vi "离线数据源.vi"(11 "显示前面板":bool) -> (0 "前面板打开":bool, 1 "电流":dbl[](array[numeric]), 2 "电压数据":dbl[](array[numeric]), 3 "脉冲数据":u32[](array[numeric]))   [LabVIEW 2020]
uses:
  <vilib>/Analysis/baseanly.llb/Mean (DBL).vi
  TCPModbus_MasterClient/MB Ethernet Master Query Read Input Registers (poly).vi
  <vilib>/Analysis/NI_AALBase.lvlib
panel:
  in  "噪声比例":dbl(knob)=0.01 min=0.01 max=0.99 step=0.01 scale=0.01..0.99 scale format="%#.2f"
  in  "加载白噪声":bool
  in  "P2-7":u16(ring)=1 items=["源量程计数CPS", "中间量程电流A", "棒位STEP", "温度(摄氏度)", "硼浓度PPM", "P2电压信号"]
  in  "P2-6":u16(ring)=1 items=["源量程计数CPS", "中间量程电流A", "棒位STEP", "温度(摄氏度)", "硼浓度PPM", "P2电压信号"]
  in  "P2-8":u16(ring) items=["源量程计数CPS", "中间量程电流A", "棒位STEP", "温度(摄氏度)", "硼浓度PPM", "P2电压信号"]
  in  "P2-5":u16(ring)=4 items=["源量程计数CPS", "中间量程电流A", "棒位STEP", "温度(摄氏度)", "硼浓度PPM", "P2电压信号"]
  in  "P2-4":u16(ring)=3 items=["源量程计数CPS", "中间量程电流A", "棒位STEP", "温度(摄氏度)", "硼浓度PPM", "P2电压信号"]
  in  "P2-3":u16(ring)=5 items=["源量程计数CPS", "中间量程电流A", "棒位STEP", "温度(摄氏度)", "硼浓度PPM", "P2电压信号"]
  in  "P2-2":u16(ring)=2 items=["源量程计数CPS", "中间量程电流A", "棒位STEP", "温度(摄氏度)", "硼浓度PPM", "P2电压信号"]
  in  "P2-6":dbl=3e-12
  in  "P2-5":dbl=500.0
  in  "P2-4":dbl=275.0
  in  "P2-3":dbl
  in  "P2-1":u16(ring)=2 items=["源量程计数CPS", "中间量程电流A", "棒位STEP", "温度(摄氏度)", "硼浓度PPM", "P2电压信号"]
  out "TCP Connection":refnum<k5>
  in  "网络端口":u16=502
  in  "网络连接IP地址":string="192.168.1.66"
  in  "网络数据源开":bool
  in  "网络数据源开关":bool
  in  "1-5V":bool
  out "Vin8":dbl format="%#_5g"
  out "Vin7":dbl format="%#_5g"
  out "Vin6":dbl format="%#_5g"
  out "Vin5":dbl format="%#_5g"
  out "Vin4":dbl format="%#_5g"
  out "Vin3":dbl format="%#_5g"
  out "Vin2":dbl format="%#_5g"
  out "Vin1":dbl format="%#_5g"
  in  "电流通道2":dbl=2e-11
  in  "电流通道1":dbl=1e-11
  in  "P2-8":dbl=1.0
  in  "P2-7":dbl=4e-12
  in  "P2-2":dbl
  in  "P2-1":dbl
  in  "脉冲3":u32=300
  in  "脉冲2":u32=200
  in  "脉冲1":u32=100
  # "CPS"
  # "A"
  # "CPS"
  # "A"
  # "CPS"
  # "0-10V"
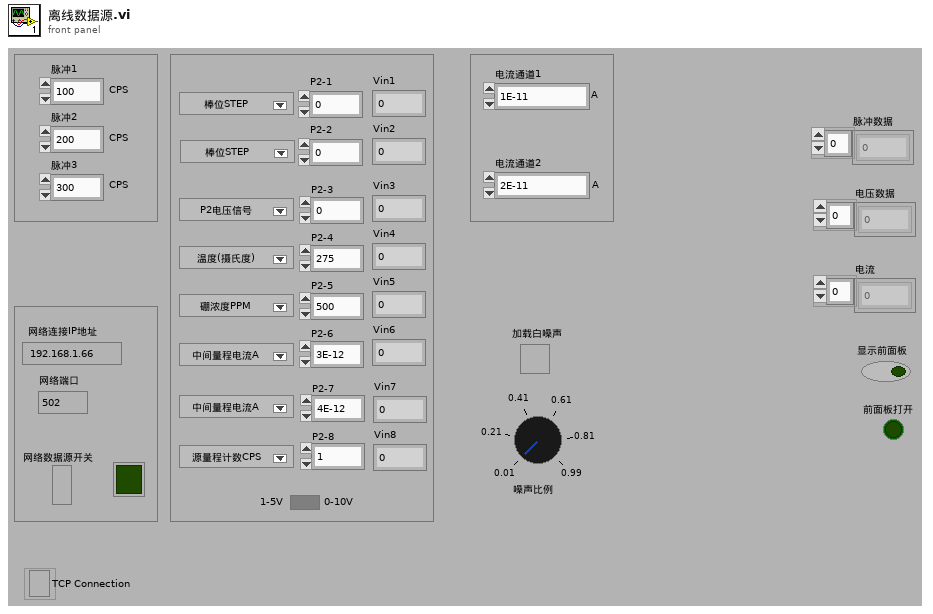
[diagram p1: front panel]
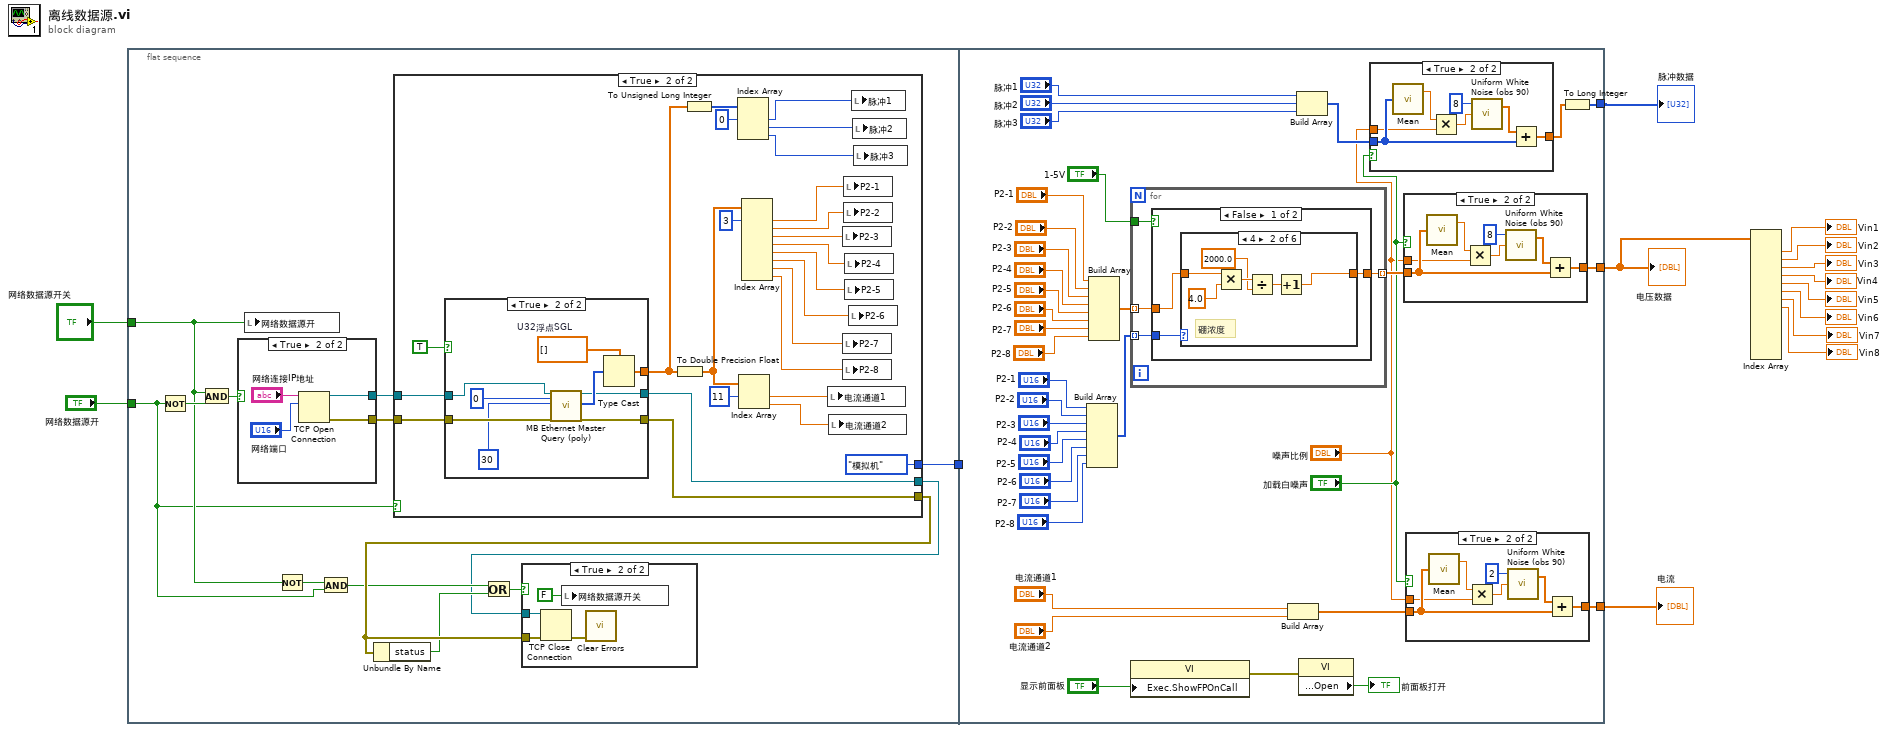
[diagram p0: block diagram]
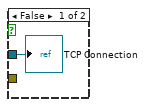
[diagram p2: hidden frame]
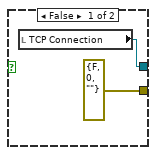
[diagram p3: hidden frame]
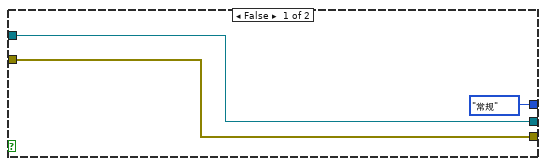
[diagram p4: hidden frame]
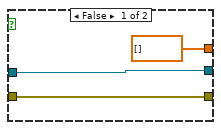
[diagram p5: hidden frame]
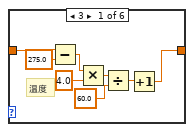
[diagram p9: hidden frame]
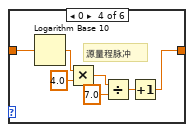
[diagram p11: hidden frame]
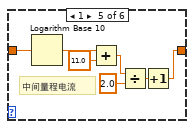
[diagram p12: hidden frame]
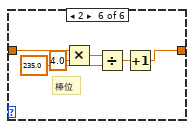
[diagram p13: hidden frame]
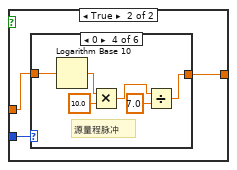
[diagram p14: hidden frame]
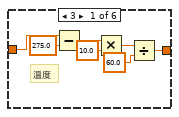
[diagram p15: hidden frame]
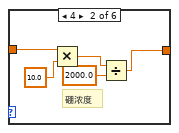
[diagram p16: hidden frame]
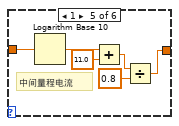
[diagram p18: hidden frame]
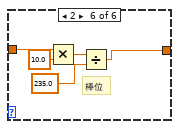
[diagram p19: hidden frame]
diagram:
  n1 = flat-sequence {
    tunnel: "网络数据源开关" -> [w24]
    tunnel: [w27] -> w13
    tunnel: "网络数据源开" -> [w22]
    tunnel: [w85] -> w3
    tunnel: [w87] -> w1
    tunnel: [w82] -> w2
    tunnel: w13 -> [_]
    frame #0 {
      n2 = Not(x=w22) -> (.not. x?=w26:bool)
      n3 = And(x=w24, y=w26) -> (x .and. y?=w25:bool)
      n4 = case shown="True" w25 {
        tunnel: [w33 w36] -> w21
        tunnel: [errorcluster {"status"=FALSE, "code"=0, "source"=""} ("error out") w35] -> w20
        frame False {
          n5 = local read "TCP Connection"() -> (w33:refnum<k5>)
        }
        frame True {
          n6 = TCP Open Connection(address="网络连接IP地址", remote port or service name="网络端口") -> (connection ID=w36:refnum<k5>, error out=w35:errorcluster)  [unwired: 1 in, 2 out]
        }
      }
      n7 = local write "网络数据源开"(w24) -> ()
      n8 = Not(x=w24) -> (.not. x?=w23:bool)
      n9 = And(x=w23, y=w22) -> (x .and. y?=w18:bool)
      n10 = case shown="True" w22 {
        tunnel: [enum32{"常规", "模拟机"}."常规" ("选项") enum32{"常规", "模拟机"}."模拟机" ("选项")] -> w27
        tunnel: w21 -> [w40 w52]
        tunnel: w20 -> [w39 w51]
        tunnel: [w39 w48] -> w19
        tunnel: [w40 w49] -> w15
        frame False {
        }
        frame True {
          n11 = case shown="True" TRUE {
            tunnel: w52 -> [w69 w75]
            tunnel: w51 -> [w68 w74]
            tunnel: [w69 w72] -> w49
            tunnel: [w68 w71] -> w48
            tunnel: [sgl[] [] ("U32浮点SGL") w70] -> w46
            frame False {
            }
            frame True {
              w76 = sgl[] []  # U32浮点SGL
              n12 = call-poly "MB Ethernet Master Query (poly).vi"("TCP Connection Refnum in"=w75, "Starting Address"=u16 0, "Quantity"=u16 30, "error in"=w74) -> ("TCP Connection Refnum (dup)"=w72:refnum<k5>, "Input Registers"=w77:u16[], "error out"=w71:errorcluster)  [unwired: 1 in, 12 out]
              n13 = Type Cast(type=w76, x=w77) -> (*(type *) &x=w70:sgl[])
            }
          }
          n14 = To Double Precision Float(number=w46) -> (double precision float=w45:dbl[])
          n15 = To Unsigned Long Integer(number=w46) -> (unsigned 32bit integer=w47:u32[])
          n16 = Index Array(array=w47, index #1=0 ("索引")) -> (element #1=w66:u32, element #2=w65:u32, element #3=w64:u32)  [unwired: 2 in]
          n17 = Index Array(array=w45, index #1=11 ("索引")) -> (element #1=w55:dbl, element #2=w54:dbl)  [unwired: 1 in]
          n18 = Index Array(array=w45, index #1=3 ("索引")) -> (element #1=w63:dbl, element #2=w62:dbl, element #3=w61:dbl, element #4=w60:dbl, element #5=w59:dbl, element #6=w58:dbl, element #7=w57:dbl, element #8=w56:dbl)  [unwired: 7 in]
          n19 = local write "电流通道1"(w55) -> ()
          n20 = local write "电流通道2"(w54) -> ()
          n21 = local write "P2-3"(w61) -> ()
          n22 = local write "P2-7"(w57) -> ()
          n23 = local write "P2-8"(w56) -> ()
          n24 = local write "P2-1"(w63) -> ()
          n25 = local write "P2-2"(w62) -> ()
          n26 = local write "P2-4"(w60) -> ()
          n27 = local write "P2-5"(w59) -> ()
          n28 = local write "P2-6"(w58) -> ()
          n29 = local write "脉冲1"(w66) -> ()
          n30 = local write "脉冲2"(w65) -> ()
          n31 = local write "脉冲3"(w64) -> ()
        }
      }
      n32 = Unbundle By Name(w19) -> ("status"=w17:bool)
      n33 = Or(x=w18, y=w17) -> (x .or. y?=w16:bool)
      n34 = case shown="True" w16 {
        tunnel: w19 -> [_ w31]
        tunnel: w15 -> [w28 w32]
        frame False {
          "TCP Connection" <- w28
        }
        frame True {
          n35 = TCP Close Connection(connection ID=w32, error in (no error)=w31) -> (error out=w30:errorcluster)  [unwired: 2 out]
          n36 = local write "网络数据源开关"(FALSE ("网络数据源开关")) -> ()
          n37 = call <vilib>:"Clear Errors.vi"("error in (no error)"=w30) -> ()  [unwired: 5 in, 2 out]
        }
      }
    }
    frame #1 {
      n38 = Build Array("P2-1", "P2-2", "P2-3", "P2-4", "P2-5", "P2-6", "P2-7", "P2-8") -> (w89:u16[])
      n39 = Build Array("P2-1", "P2-2", "P2-3", "P2-4", "P2-5", "P2-6", "P2-7", "P2-8") -> (w99:dbl[])
      n40 = for {
        tunnel: w99 -> [w141] mode=indexing
        tunnel: [w140] -> w84 mode=indexing
        tunnel: "1-5V" -> [w142]
        tunnel: w89 -> [w139] mode=indexing
        n41 = case shown="False" w142 {
          tunnel: w141 -> [w145 w183]
          tunnel: [w144 w182] -> w140
          tunnel: w139 -> [w143 w181]
          frame False {
            n42 = case shown="4" w143 {
              tunnel: w145 -> [w148 w159 w160 w163 w170 w177]
              tunnel: [w146 w154 w160 w161 w168 w175] -> w144
              frame 3 {
                # "温度"
                n43 = Subtract(x=w148, y=275.0) -> (x-y=w149:dbl)
                n44 = Multiply(x=w149, y=4.0) -> (x*y=w151:dbl)
                n45 = Divide(x=w151, y=60.0) -> (x/y=w147:dbl)
                n46 = Increment(x=w147) -> (x+1=w146:dbl)
              }
              frame 4 {
                # "硼浓度"
                n47 = Multiply(x=w159, y=4.0) -> (x*y=w157:dbl)
                n48 = Divide(x=w157, y=2000.0) -> (x/y=w155:dbl)
                n49 = Increment(x=w155) -> (x+1=w154:dbl)
              }
              frame Default {
              }
              frame 0 {
                # "源量程脉冲"
                n50 = Logarithm Base 10(1:w163) -> (0:w164:dbl)
                n51 = Multiply(x=w164, y=4.0) -> (x*y=w167:dbl)
                n52 = Divide(x=w167, y=7.0) -> (x/y=w162:dbl)
                n53 = Increment(x=w162) -> (x+1=w161:dbl)
              }
              frame 1 {
                # "中间量程电流"
                n54 = Logarithm Base 10(1:w170) -> (0:w171:dbl)
                n55 = Add(x=w171, y=11.0) -> (x+y=w174:dbl)
                n56 = Divide(x=w174, y=2.0) -> (x/y=w169:dbl)
                n57 = Increment(x=w169) -> (x+1=w168:dbl)
              }
              frame 2 {
                # "棒位"
                n58 = Multiply(x=w177, y=4.0) -> (x*y=w179:dbl)
                n59 = Divide(x=w179, y=235.0) -> (x/y=w176:dbl)
                n60 = Increment(x=w176) -> (x+1=w175:dbl)
              }
            }
          }
          frame True {
            n61 = case shown="0" w181 {
              tunnel: w183 -> [w185 w195 w196 w198 w204 w210]
              tunnel: [w184 w191 w196 w197 w203 w209] -> w182
              frame 3 {
                # "温度"
                n62 = Subtract(x=w185, y=275.0) -> (x-y=w186:dbl)
                n63 = Multiply(x=w186, y=10.0) -> (x*y=w188:dbl)
                n64 = Divide(x=w188, y=60.0) -> (x/y=w184:dbl)
              }
              frame 4 {
                # "硼浓度"
                n65 = Multiply(x=w195, y=10.0) -> (x*y=w193:dbl)
                n66 = Divide(x=w193, y=2000.0) -> (x/y=w191:dbl)
              }
              frame Default {
              }
              frame 0 {
                # "源量程脉冲"
                n67 = Logarithm Base 10(1:w198) -> (0:w199:dbl)
                n68 = Multiply(x=w199, y=10.0) -> (x*y=w202:dbl)
                n69 = Divide(x=w202, y=7.0) -> (x/y=w197:dbl)
              }
              frame 1 {
                # "中间量程电流"
                n70 = Logarithm Base 10(1:w204) -> (0:w205:dbl)
                n71 = Add(x=w205, y=11.0) -> (x+y=w208:dbl)
                n72 = Divide(x=w208, y=0.8) -> (x/y=w203:dbl)
              }
              frame 2 {
                # "棒位"
                n73 = Multiply(x=w210, y=10.0) -> (x*y=w212:dbl)
                n74 = Divide(x=w212, y=235.0) -> (x/y=w209:dbl)
              }
            }
          }
        }
      }
      n75 = property class="VI"("Exec.ShowFPOnCall"="显示前面板") -> (error out=w112:errorcluster)  [unwired: 2 in, 1 out]
      n76 = Build Array("电流通道1", "电流通道2") -> (w86:dbl[])
      n77 = Build Array("脉冲1", "脉冲2", "脉冲3") -> (w83:u32[])
      n78 = property class="VI"(error in=w112) -> ("Front Panel.Open"=→"前面板打开":bool)  [unwired: 1 in, 2 out]
      n79 = case shown="True" "加载白噪声" {
        tunnel: [w115 w121] -> w81
        tunnel: w83 -> [w115 w119]
        tunnel: "噪声比例" -> [_ w116]
        frame False {
        }
        frame True {
          n80 = call-poly <vilib>:"Mean.vi"("X"=w119) -> ("mean"=w118:dbl)  [unwired: 1 out]
          n81 = Multiply(x=w118, y=w116) -> (x*y=w117:dbl)
          n82 = call <vilib>:"Uniform White Noise (obs 90).vi"("amplitude"=w117, "samples"=8) -> ("uniform white noise"=w120:dbl[])  [unwired: 1 in, 1 out]
          n83 = Add(x=w120, y=w119) -> (x+y=w121:dbl[])
        }
      }
      n84 = case shown="True" "加载白噪声" {
        tunnel: [w123 w129] -> w85
        tunnel: w84 -> [w123 w127]
        tunnel: "噪声比例" -> [_ w124]
        frame False {
        }
        frame True {
          n85 = call-poly <vilib>:"Mean.vi"("X"=w127) -> ("mean"=w126:dbl)  [unwired: 1 out]
          n86 = Multiply(x=w126, y=w124) -> (x*y=w125:dbl)
          n87 = call <vilib>:"Uniform White Noise (obs 90).vi"("amplitude"=w125, "samples"=8) -> ("uniform white noise"=w128:dbl[])  [unwired: 1 in, 1 out]
          n88 = Add(x=w128, y=w127) -> (x+y=w129:dbl[])
        }
      }
      n89 = case shown="True" "加载白噪声" {
        tunnel: [w131 w137] -> w87
        tunnel: w86 -> [w131 w135]
        tunnel: "噪声比例" -> [_ w132]
        frame False {
        }
        frame True {
          n90 = call-poly <vilib>:"Mean.vi"("X"=w135) -> ("mean"=w134:dbl)  [unwired: 1 out]
          n91 = Multiply(x=w134, y=w132) -> (x*y=w133:dbl)
          n92 = call <vilib>:"Uniform White Noise (obs 90).vi"("amplitude"=w133, "samples"=2) -> ("uniform white noise"=w136:dbl[])  [unwired: 1 in, 1 out]
          n93 = Add(x=w136, y=w135) -> (x+y=w137:dbl[])
        }
      }
      n94 = To Long Integer(number=w81) -> (32bit integer=w82:i32[])
    }
  }
  n95 = Index Array(array=w3) -> (element #1=→"Vin1":dbl, element #2=→"Vin2":dbl, element #3=→"Vin3":dbl, element #4=→"Vin4":dbl, element #5=→"Vin5":dbl, element #6=→"Vin6":dbl, element #7=→"Vin7":dbl, element #8=→"Vin8":dbl)  [unwired: 14 in, 6 out]
  "脉冲数据" <- w2
  "电压数据" <- w3
  "电流" <- w1
